vi "Dashboard Main.vi"() -> ()   [LabVIEW 2013]
uses:
  frc 2014 Vision Prototype/TargetType.ctl
  <vilib>/event_ctls.llb/eventvkey.ctl
  <vilib>/Analysis/baseanly.llb/Mean (DBL).vi
  <vilib>/Rock Robotics/WPI/Dashboard/WPI_DashboardLogging Global.vi
  <vilib>/Utility/config.llb/Write Key (String).vi
  <vilib>/Utility/config.llb/Write Key (I32).vi
  <vilib>/Utility/config.llb/NI_LVConfig.lvlib
  <vilib>/Analysis/NI_AALBase.lvlib
panel:
  out "Camera IP":string="10.15.72.11"
  out "Raw Distance":dbl[](array[numeric]) format="%#.4g"
  out "Error":bool
  out "Mask":T1(plugin-control)
  out "Target Info":T3(array[cluster])
  in  "Camera Type":enum16{"206", "1011", "1013"}(ring)=enum."1011"
  in  "Std Devs":cluster{"Hue":dbl, "Sat":dbl, "Val":dbl}={"Hue"=4.0, "Sat"=6.0, "Val"=4.0}
  out "x":dbl
  in  "Vision_Control":u8(slide) scale=0.0..2.0
  in  "Camera Settings":T4={"Frame Rate"=30, "Compression"=30, "Size"=1} {"Frame Rate" scale=1.0..30.0; "Size" items=["640x480", "320x240", "160x120"]}
  out "Image Message":string="Timeout in Camera Communications"
  in  "Rec Mode":enum32{"Stop", "Record", "Playback"}(radio)
  in  "Dashboard Tab":T5(tab)
  out "MotorSliders R":cluster{"MotorSlide1":dbl, "MotorSlide2":dbl} {"MotorSlide2" scale=-1.0..1.0 scale format="%#_2e"; "MotorSlide1" scale=-1.0..1.0 scale format="%#_2e"}
  out "MotorChart R":cluster{"Numeric":dbl, "Numeric":dbl}(graph)
  out "MotorSliders L":T6 {"MotorSlide4 2" scale=0.0..14.0 scale format="%#_2e"; "MotorSlide2" scale=-1.0..1.0 scale format="%#_2e"; "MotorSlide1" scale=-1.0..1.0 scale format="%#_2e"}
  out "MotorChart L":T7(graph)
  out "JS1 Z":dbl(slide) scale=-1.0..1.0 scale format="%#_2e"
  out "Joystick 1":cluster{"X":dbl, "Y":dbl}[](graph)
  out "JS Buttons 1":T8
  out "JS2 Z":dbl(slide) scale=-1.0..1.0 scale format="%#_2e"
  out "Joystick 2":cluster{"X":dbl, "Y":dbl}[](graph)
  out "JS Buttons 2":T8
  out "Mode":T9(ring)=enum."Auto Disabled"
  in  "DB Camera Config":bool
  out "fps":dbl format="%#.1g"
  out "Mbps":dbl format="%#.1g"
  out "Mbps 2":bool
  out "LED 1":bool
  out "Compressor_Running":bool
  out "Shooter_State":string
  out "Hot_Target_Angle":dbl(knob) scale=-90.0..90.0
  out "Target_Left_Hot":bool
  out "units 2":string="feet"
  out "vision_target_distance":dbl(slide) caption="sonar_distance" scale=0.0..25.0 scale format="%#.3g"
  out "units":string="inches"
  out "sonar_ball_distance":dbl(slide) caption="sonar_distance" scale=0.0..120.0 scale format="%#.3g"
  out "robot_heading":dbl(knob) scale=0.0..360.0
  out "Target_Right_Hot":bool
  in  "Dist_Fifo":i32=5
  in  "Color Components":T10={"Hue"={100.0, 190.0}, "Sat"={121.42857142857142, 255.0}, "Val"={188.2142857142857, 255.0}} {"Val" scale=0.0..255.0; "Sat" scale=0.0..255.0; "Hue" scale=0.0..255.0 scale format="%#_3g"}
  in  "Area Size Limit %":dbl=0.06 format="%#_13g"
  in  "Score Cutoff":dbl(slide)=54.248366013071895 scale=0.0..100.0
  in  "Fudge Factor":dbl=-1.0
  in  "Scale Factor Adustment":dbl
  out "Median \nDistance":dbl
  out "Final Target Dist From Center":dbl
  out "Final Target\nDistance":dbl
  in  "Test Slider":dbl(slide) scale=0.0..100.0 scale format="%#_3g"
  in  "On/Off":bool caption="Solenoid"
  in  "Test Name":u16(ring) items=["Select the test to run...", "Example Test", "-------------------------------", "List of tests is built in robot code.", "Replace with your own automated tests."]
  in  "Test Tree":string(tree)
  in  "Motor":cluster{"Value":dbl, "Enable":bool} {"Value" scale=-1.0..1.0 scale format="%#_3g"}
  out "Progress":T11 {"Test Progress" scale=0.0..100.0}
  in  "Rev/Fwd":cluster{"Forward":bool, "Reverse":bool}
  in  "Test Ring":u16(ring) items=["Auto", "Fixed indoor", "Fixed outdoor 1", "Fixed outdoor 2", "Fixed fluorescent 1", "Fixed fluorescent 2", "Hold current"]
  in  "Listbox":i32(listbox)
  out "Tree":string(tree)
  out "Camera Image":T1(plugin-control)
  # "Left"
  # "Front"
  # "Right"
  # "Battery"
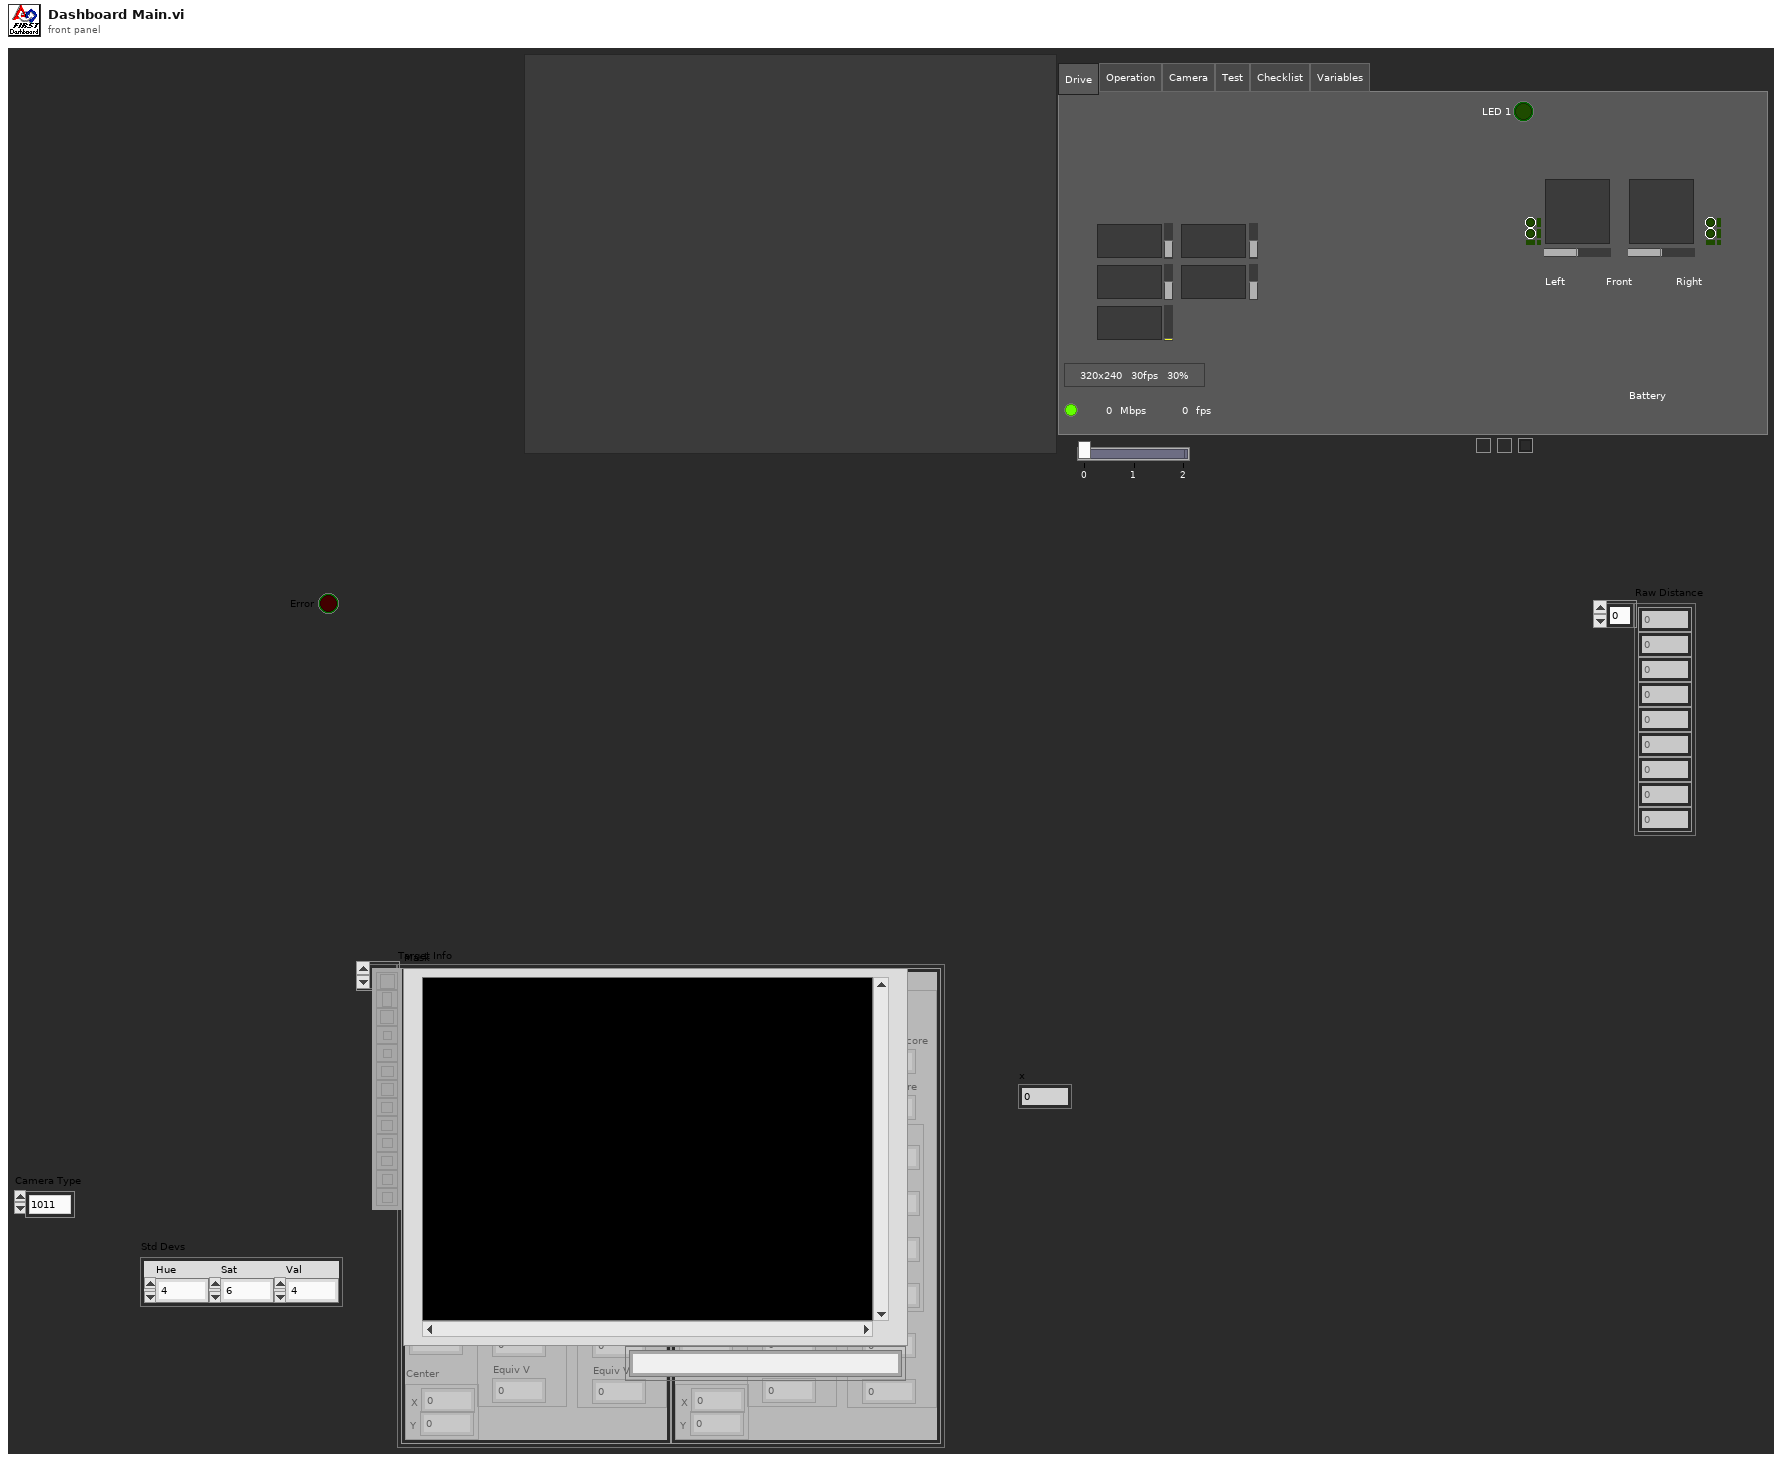
[diagram p1: front panel]
types:
  T1 = typedef "IMAQ Image.ctl" = refnum<image>
  T2 = typedef "TargetType.ctl" = enum16{"Not Hot", "Hot"}
  T3 = cluster{"Scores":cluster{"Total":dbl, "Left":dbl, "Right":dbl, "Ratio":dbl, "Vertical":dbl, "index":i32, "State":T2}, "Verticals":cluster{"Horizontal?":bool, "Aspect Score":dbl, "Rect Score":dbl, cluster{"Left":dbl, "Top":dbl, "Right":dbl, "Bottom":dbl}, "Equiv H":dbl, "Equiv V":dbl}, "Horizontals":cluster{"Horizontal?":bool, "Aspect Score":dbl, "Rect Score":dbl, cluster{"Left":dbl, "Top":dbl, "Right":dbl, "Bottom":dbl}, "Equiv H":dbl, "Equiv V":dbl}, "Distance ft":dbl, "Center":cluster{"X":dbl, "Y":dbl}}[]
  T4 = cluster{"Frame Rate":i32, "Compression":i32, "Size":u16}
  T5 = enum32{"Drive", "Operation", "Camera", "Test", "Checklist", "Variables"}
  T6 = cluster{"MotorSlide1":dbl, "MotorSlide2":dbl, "MotorSlide4 2":dbl}
  T7 = cluster{"Numeric":dbl, "Numeric":dbl, "Battery":sgl}
  T8 = cluster{bool, bool, bool, bool, bool, bool, bool, bool, bool, bool, bool, bool}
  T9 = enum8{"Tele-Op Disabled", "Tele-Op Enabled", "Auto Disabled", "Auto Enabled", "Test Disabled", "Test Enabled", ""}
  T10 = cluster{"Hue":cluster{dbl, dbl}, "Sat":cluster{dbl, dbl}, "Val":cluster{dbl, dbl}}
  T11 = cluster{"Test Progress":u8, "Test Progress Text":string}
  T12 = enum32{"Drive", "Operation", "Auto", "Test", "Checklist", "Variables"}
  T13 = typedef "Image Type" = u32
  T14 = cluster{"Horizontal":bool, "Aspect Score":dbl, "Rect Score":dbl, cluster{"Left":dbl, "Top":dbl, "Right":dbl, "Bottom":dbl}, "Equiv H":dbl, "Equiv V":dbl}[]
  T15 = cluster{cluster{dbl, dbl}, cluster{dbl, dbl}, cluster{dbl, dbl}}
  T16 = cluster{"Scores":cluster{"Total":dbl, "Left":dbl, "Right":dbl, "Ratio":dbl, "Vertical":dbl, "index":i32, "State":T2}, "Verticals":cluster{"Horizontal?":bool, "Aspect Score":dbl, "Rect Score":dbl, cluster{"Left":dbl, "Top":dbl, "Right":dbl, "Bottom":dbl}, "Equiv H":dbl, "Equiv V":dbl}, "Horizontals":cluster{"Horizontal?":bool, "Aspect Score":dbl, "Rect Score":dbl, cluster{"Left":dbl, "Top":dbl, "Right":dbl, "Bottom":dbl}, "Equiv H":dbl, "Equiv V":dbl}, "Validated":bool}[]
  T17 = cluster{"Distance (ft)":dbl, "Target Center (-1 to 1)":cluster{"X":dbl, "Y":dbl}, "Left":bool, "State":T2}[]
  T18 = cluster{"Scores":cluster{"Total":dbl, "Left":dbl, "Right":dbl, "Ratio":dbl, "Vertical":dbl, "index":i32, "State":T2}, "Verticals":cluster{"Horizontal?":bool, "Aspect Score":dbl, "Rect Score":dbl, cluster{"Left":dbl, "Top":dbl, "Right":dbl, "Bottom":dbl}, "Equiv H":dbl, "Equiv V":dbl}, "Horizontals":cluster{"Horizontal?":bool, "Aspect Score":dbl, "Rect Score":dbl, cluster{"Left":dbl, "Top":dbl, "Right":dbl, "Bottom":dbl}, "Equiv H":dbl, "Equiv V":dbl}, "Distance (ft)":dbl, "Target Center (-1 to 1)":cluster{"X":dbl, "Y":dbl}}[]
  T19 = cluster{"Distances[0]":cluster{"Distance (ft)":dbl, "Target Center (-1 to 1)":cluster{"X":dbl, "Y":dbl}, "Left":bool, "State":T2}, "Distances[1]":cluster{"Distance (ft)":dbl, "Target Center (-1 to 1)":cluster{"X":dbl, "Y":dbl}, "Left":bool, "State":T2}, "Distances[2]":cluster{"Distance (ft)":dbl, "Target Center (-1 to 1)":cluster{"X":dbl, "Y":dbl}, "Left":bool, "State":T2}, "Distances[3]":cluster{"Distance (ft)":dbl, "Target Center (-1 to 1)":cluster{"X":dbl, "Y":dbl}, "Left":bool, "State":T2}, "Distances[4]":cluster{"Distance (ft)":dbl, "Target Center (-1 to 1)":cluster{"X":dbl, "Y":dbl}, "Left":bool, "State":T2}, "Distances[5]":cluster{"Distance (ft)":dbl, "Target Center (-1 to 1)":cluster{"X":dbl, "Y":dbl}, "Left":bool, "State":T2}, "Distances[6]":cluster{"Distance (ft)":dbl, "Target Center (-1 to 1)":cluster{"X":dbl, "Y":dbl}, "Left":bool, "State":T2}, "Distances[7]":cluster{"Distance (ft)":dbl, "Target Center (-1 to 1)":cluster{"X":dbl, "Y":dbl}, "Left":bool, "State":T2}, "Distances[8]":cluster{"Distance (ft)":dbl, "Target Center (-1 to 1)":cluster{"X":dbl, "Y":dbl}, "Left":bool, "State":T2}}
  T20 = cluster{"Target Info[0]":cluster{"Scores":cluster{"Total":dbl, "Left":dbl, "Right":dbl, "Ratio":dbl, "Vertical":dbl, "index":i32, "State":T2}, "Verticals":cluster{"Horizontal?":bool, "Aspect Score":dbl, "Rect Score":dbl, cluster{"Left":dbl, "Top":dbl, "Right":dbl, "Bottom":dbl}, "Equiv H":dbl, "Equiv V":dbl}, "Horizontals":cluster{"Horizontal?":bool, "Aspect Score":dbl, "Rect Score":dbl, cluster{"Left":dbl, "Top":dbl, "Right":dbl, "Bottom":dbl}, "Equiv H":dbl, "Equiv V":dbl}, "Distance (ft)":dbl, "Target Center (-1 to 1)":cluster{"X":dbl, "Y":dbl}}, "Target Info[1]":cluster{"Scores":cluster{"Total":dbl, "Left":dbl, "Right":dbl, "Ratio":dbl, "Vertical":dbl, "index":i32, "State":T2}, "Verticals":cluster{"Horizontal?":bool, "Aspect Score":dbl, "Rect Score":dbl, cluster{"Left":dbl, "Top":dbl, "Right":dbl, "Bottom":dbl}, "Equiv H":dbl, "Equiv V":dbl}, "Horizontals":cluster{"Horizontal?":bool, "Aspect Score":dbl, "Rect Score":dbl, cluster{"Left":dbl, "Top":dbl, "Right":dbl, "Bottom":dbl}, "Equiv H":dbl, "Equiv V":dbl}, "Distance (ft)":dbl, "Target Center (-1 to 1)":cluster{"X":dbl, "Y":dbl}}, "Target Info[2]":cluster{"Scores":cluster{"Total":dbl, "Left":dbl, "Right":dbl, "Ratio":dbl, "Vertical":dbl, "index":i32, "State":T2}, "Verticals":cluster{"Horizontal?":bool, "Aspect Score":dbl, "Rect Score":dbl, cluster{"Left":dbl, "Top":dbl, "Right":dbl, "Bottom":dbl}, "Equiv H":dbl, "Equiv V":dbl}, "Horizontals":cluster{"Horizontal?":bool, "Aspect Score":dbl, "Rect Score":dbl, cluster{"Left":dbl, "Top":dbl, "Right":dbl, "Bottom":dbl}, "Equiv H":dbl, "Equiv V":dbl}, "Distance (ft)":dbl, "Target Center (-1 to 1)":cluster{"X":dbl, "Y":dbl}}, "Target Info[3]":cluster{"Scores":cluster{"Total":dbl, "Left":dbl, "Right":dbl, "Ratio":dbl, "Vertical":dbl, "index":i32, "State":T2}, "Verticals":cluster{"Horizontal?":bool, "Aspect Score":dbl, "Rect Score":dbl, cluster{"Left":dbl, "Top":dbl, "Right":dbl, "Bottom":dbl}, "Equiv H":dbl, "Equiv V":dbl}, "Horizontals":cluster{"Horizontal?":bool, "Aspect Score":dbl, "Rect Score":dbl, cluster{"Left":dbl, "Top":dbl, "Right":dbl, "Bottom":dbl}, "Equiv H":dbl, "Equiv V":dbl}, "Distance (ft)":dbl, "Target Center (-1 to 1)":cluster{"X":dbl, "Y":dbl}}, "Target Info[4]":cluster{"Scores":cluster{"Total":dbl, "Left":dbl, "Right":dbl, "Ratio":dbl, "Vertical":dbl, "index":i32, "State":T2}, "Verticals":cluster{"Horizontal?":bool, "Aspect Score":dbl, "Rect Score":dbl, cluster{"Left":dbl, "Top":dbl, "Right":dbl, "Bottom":dbl}, "Equiv H":dbl, "Equiv V":dbl}, "Horizontals":cluster{"Horizontal?":bool, "Aspect Score":dbl, "Rect Score":dbl, cluster{"Left":dbl, "Top":dbl, "Right":dbl, "Bottom":dbl}, "Equiv H":dbl, "Equiv V":dbl}, "Distance (ft)":dbl, "Target Center (-1 to 1)":cluster{"X":dbl, "Y":dbl}}, "Target Info[5]":cluster{"Scores":cluster{"Total":dbl, "Left":dbl, "Right":dbl, "Ratio":dbl, "Vertical":dbl, "index":i32, "State":T2}, "Verticals":cluster{"Horizontal?":bool, "Aspect Score":dbl, "Rect Score":dbl, cluster{"Left":dbl, "Top":dbl, "Right":dbl, "Bottom":dbl}, "Equiv H":dbl, "Equiv V":dbl}, "Horizontals":cluster{"Horizontal?":bool, "Aspect Score":dbl, "Rect Score":dbl, cluster{"Left":dbl, "Top":dbl, "Right":dbl, "Bottom":dbl}, "Equiv H":dbl, "Equiv V":dbl}, "Distance (ft)":dbl, "Target Center (-1 to 1)":cluster{"X":dbl, "Y":dbl}}, "Target Info[6]":cluster{"Scores":cluster{"Total":dbl, "Left":dbl, "Right":dbl, "Ratio":dbl, "Vertical":dbl, "index":i32, "State":T2}, "Verticals":cluster{"Horizontal?":bool, "Aspect Score":dbl, "Rect Score":dbl, cluster{"Left":dbl, "Top":dbl, "Right":dbl, "Bottom":dbl}, "Equiv H":dbl, "Equiv V":dbl}, "Horizontals":cluster{"Horizontal?":bool, "Aspect Score":dbl, "Rect Score":dbl, cluster{"Left":dbl, "Top":dbl, "Right":dbl, "Bottom":dbl}, "Equiv H":dbl, "Equiv V":dbl}, "Distance (ft)":dbl, "Target Center (-1 to 1)":cluster{"X":dbl, "Y":dbl}}, "Target Info[7]":cluster{"Scores":cluster{"Total":dbl, "Left":dbl, "Right":dbl, "Ratio":dbl, "Vertical":dbl, "index":i32, "State":T2}, "Verticals":cluster{"Horizontal?":bool, "Aspect Score":dbl, "Rect Score":dbl, cluster{"Left":dbl, "Top":dbl, "Right":dbl, "Bottom":dbl}, "Equiv H":dbl, "Equiv V":dbl}, "Horizontals":cluster{"Horizontal?":bool, "Aspect Score":dbl, "Rect Score":dbl, cluster{"Left":dbl, "Top":dbl, "Right":dbl, "Bottom":dbl}, "Equiv H":dbl, "Equiv V":dbl}, "Distance (ft)":dbl, "Target Center (-1 to 1)":cluster{"X":dbl, "Y":dbl}}, "Target Info[8]":cluster{"Scores":cluster{"Total":dbl, "Left":dbl, "Right":dbl, "Ratio":dbl, "Vertical":dbl, "index":i32, "State":T2}, "Verticals":cluster{"Horizontal?":bool, "Aspect Score":dbl, "Rect Score":dbl, cluster{"Left":dbl, "Top":dbl, "Right":dbl, "Bottom":dbl}, "Equiv H":dbl, "Equiv V":dbl}, "Horizontals":cluster{"Horizontal?":bool, "Aspect Score":dbl, "Rect Score":dbl, cluster{"Left":dbl, "Top":dbl, "Right":dbl, "Bottom":dbl}, "Equiv H":dbl, "Equiv V":dbl}, "Distance (ft)":dbl, "Target Center (-1 to 1)":cluster{"X":dbl, "Y":dbl}}}
  T21 = cluster{"Horizontal?":bool, "Aspect Score":dbl, "Rect Score":dbl, cluster{"Left":dbl, "Top":dbl, "Right":dbl, "Bottom":dbl}, "Equiv H":dbl, "Equiv V":dbl}
  T22 = cluster{"Left":dbl, "Top":dbl, "Right":dbl, "Bottom":dbl}
  T23 = cluster{"Distance (ft)":dbl, "Left":dbl, "Right":dbl}
  T24 = cluster{"Digital Inputs":bool[], "Digital Outputs":bool[]}
  T25 = cluster{"Competition mode":bool, "Robot Link":bool, "Autonomous":bool, "Enabled":bool, "E-Stop":bool, "Simulated":bool, "TestMode":bool, "Docked Window":bool}
  T26 = cluster{"Boolean Array[0]":bool, "Boolean Array[1]":bool, "Boolean Array[2]":bool, "Boolean Array[3]":bool, "Boolean Array[4]":bool, "Boolean Array[5]":bool, "Boolean Array[6]":bool, "Boolean Array[7]":bool, "Boolean Array[8]":bool, "Boolean Array[9]":bool, "Boolean Array[10]":bool, "Boolean Array[11]":bool}
  T27 = typedef "NI_LVConfig.lvlib/Config Data RefNum.ctl" = refnum<k1>
  T28 = typedef "eventvkey.ctl" = enum16{"ASCII", "Enter", "Return", "Shift", "Ctrl", "Alt", "Cmd", "Opt", "Caps", "NumLock", "Clear", "Break", "Up", "Down", "Left", "Right", "Insert", "Delete", "Home", "End", "PageUp", "PageDown", "Escape", "Help", "Pause", "ScrollLock", "F1", "F2", "F3", "F4", "F5", "F6", "F7", "F8", "F9", "F10", "F11", "F12", "F13", "F14", "F15", "F16", "F17", "F18", "F19", "F20", "F21", "F22", "F23", "F24", "Play", "VolumeUp", "VolumeDown", "Mute", "Two Byte Char"}
  T29 = cluster{"Image Size":bool, "Image Type":bool, "Pixel Value":bool, "ROI Information":bool, "Zoom Factor":bool}
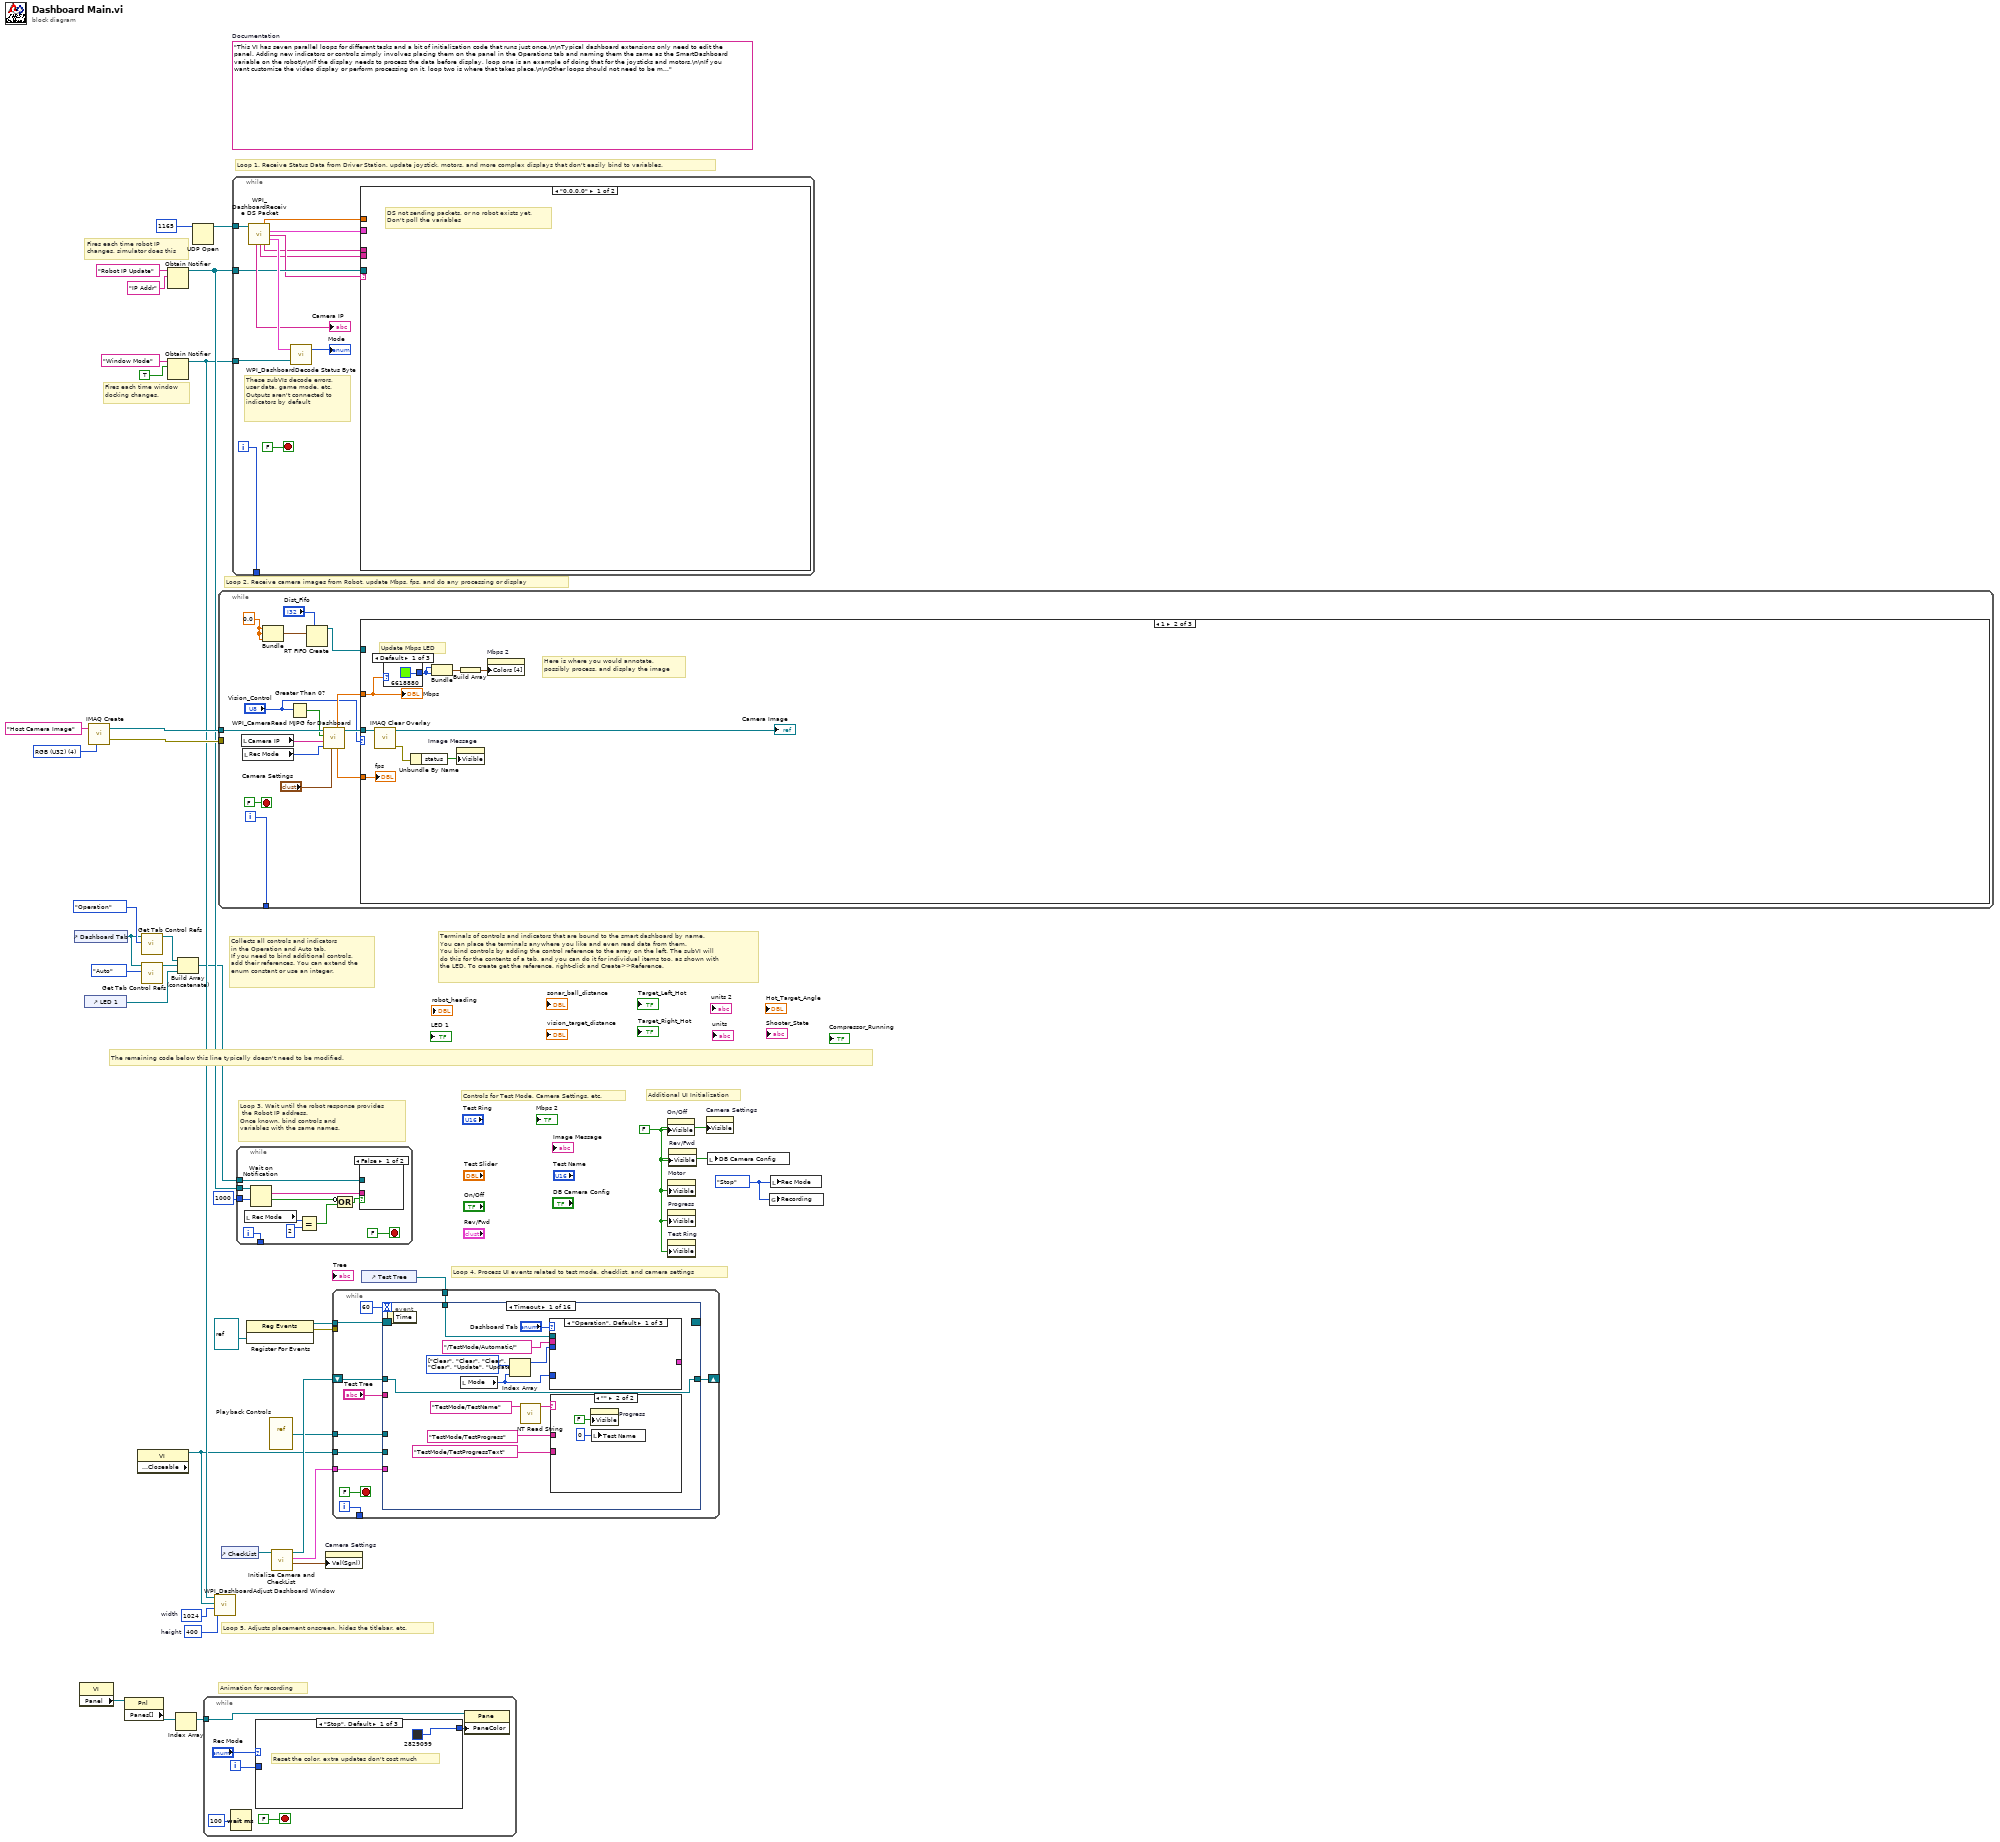
[diagram p0: block diagram]
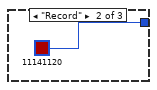
[diagram p2: hidden frame]
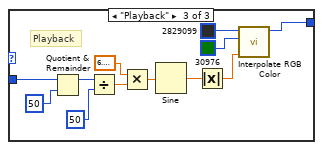
[diagram p3: hidden frame]
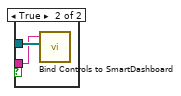
[diagram p4: hidden frame]
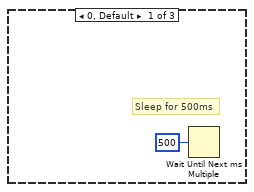
[diagram p5: hidden frame]
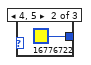
[diagram p6: hidden frame]
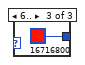
[diagram p7: hidden frame]
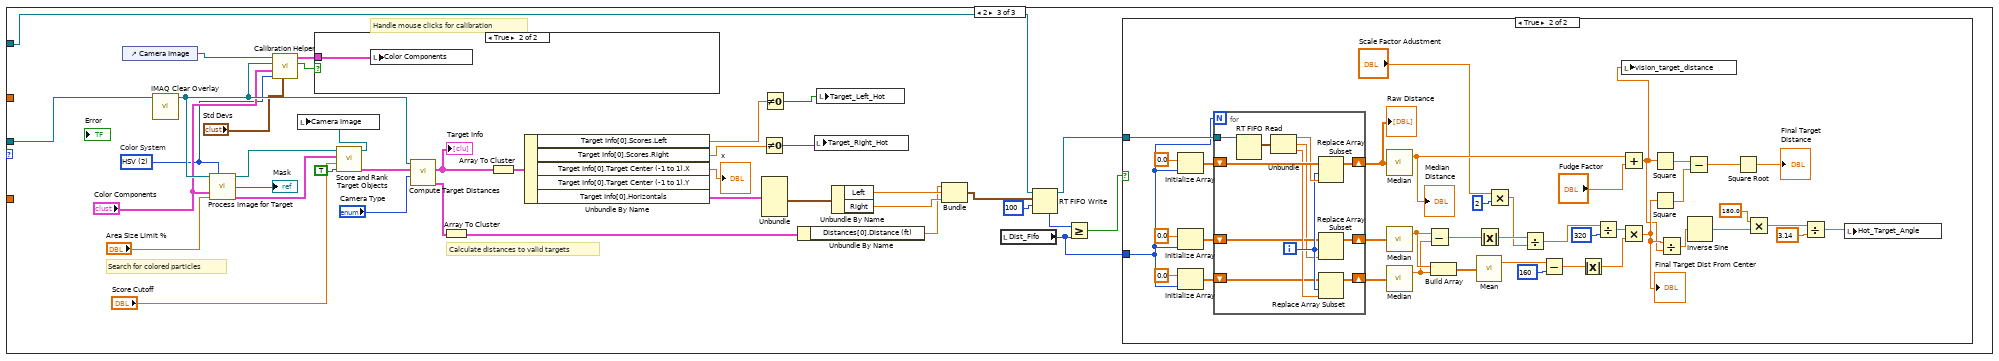
[diagram p8: hidden frame]
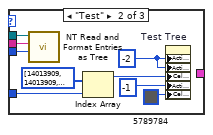
[diagram p11: hidden frame]
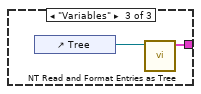
[diagram p12: hidden frame]
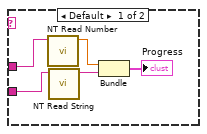
[diagram p13: hidden frame]
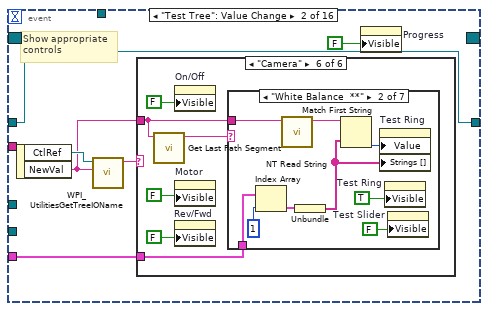
[diagram p14: hidden frame]
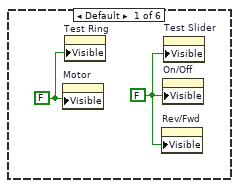
[diagram p15: hidden frame]
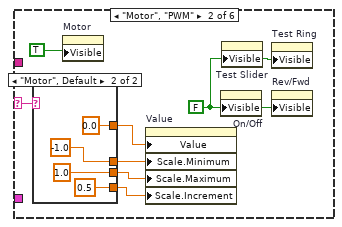
[diagram p16: hidden frame]
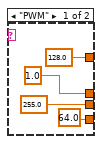
[diagram p17: hidden frame]
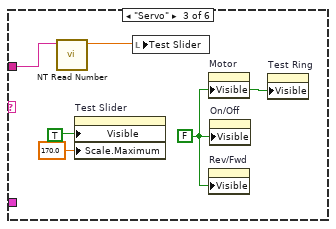
[diagram p18: hidden frame]
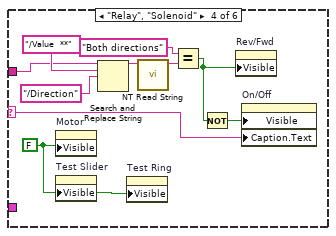
[diagram p19: hidden frame]
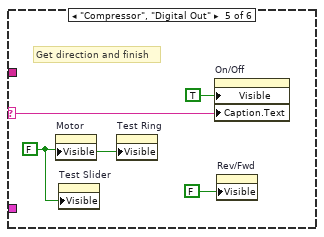
[diagram p20: hidden frame]
diagram:
  w8 = enum32{"Stop", "Record", "Playback"}."Stop" ("Rec Mode")
  w11 = 400  # height
  w12 = 1024  # width
  w25 = FALSE ("Visible")
  (unwired) "This VI has seven parallel loops for different tasks and a bit of initialization code that runs just once.\n\nTypical dashboard extensions only need to edit the panel. Adding new indicators or controls simply involves placing them on the panel in the Operations tab and naming them the same as the SmartDashboard variable on the robot\n\nIf the display needs to process the data before display, loop one is an example of doing that for the joysticks and motors.\n\nIf you want customize the video display or perform processing on it, loop two is where that takes place.\n\nOther loops should not need to be modified. They are pretty standard, and document the task they perform."  # Documentation
  w35 = T13 4 items=["Grayscale (U8)", "Grayscale (I16)", "Grayscale (SGL)", "Complex (CSG)", "RGB (U32)", "HSL (U32)", "RGB (U64)"] ("Image Type")
  # "Controls for Test Mode, Camera Settings, etc."
  # "Additional UI Initialization"
  # "Animation for recording"
  # "Fires each time robot IP\nchanges, simulator does this"
  # "Fires each time window\ndocking changes."
  # "Collects all controls and indicators\nin the Operation and Auto tab.\nIf you need to bind additional controls,\nadd their references. You can extend the\nenum constant or use an integer."
  # "The remaining code below this line typically doesn't need to be modified."
  # "Loop 4. Process UI events related to test mode, checklist, and camera settings"
  # "Terminals of controls and indicators that are bound to the smart dashboard by name.\nYou can place the terminals anywhere you like and even read data from them.\nYou bind controls by adding the control reference to the array on the left. The subVI will\ndo this for the contents of a tab, and you can do it for individual items too, as shown with\nthe LED. To create get the reference, right-click and Create>>Reference."
  # "Loop 3. Wait until the robot response provides\n the Robot IP address.\nOnce known, bind controls and\nvariables with the same names."
  # "Loop 5. Adjusts placement onscreen, hides the titlebar, etc."
  # "Loop 1. Receive Status Data from Driver Station, update joystick, motors, and more complex displays that don't easily bind to variables."
  # "Loop 2. Receive camera images from Robot, update Mbps, fps, and do any processing or display"
  n1 = control-ref of="Dashboard Tab"() -> (w6:refnum<vi>)
  n2 = property class="VI"() -> ("Panel"=w19:refnum<vi>)  [unwired: 2 in, 2 out]
  n3 = control-ref of="LED 1"() -> (w1:refnum<vi>)
  n4 = call "IMAQ Create"("Image Name"="Host Camera Image", "Image Type"=w35) -> ("New Image"=w33:T1, "error out"=w32:errorcluster)  [unwired: 2 in, 1 out]
  n5 = property class="Pnl"(reference=w19) -> ("Panes[]"=w20:refnum<vi>[])  [unwired: 1 in, 2 out]
  n6 = property class="VI" props=["Front Panel.Closeable"]() -> (reference out=w7:refnum<vi>)  [unwired: 2 in, 2 out]
  n7 = call <vilib>:"Get Tab Control Refs.vi"("Page Index"=T12."Operation" ("Dashboard Tab"), "TabControl in"=w6) -> ("ControlsOnPage"=w4:refnum<vi>[])  [unwired: 9 in]
  n8 = call <vilib>:"Get Tab Control Refs.vi"("Page Index"=T12."Auto" ("Dashboard Tab"), "TabControl in"=w6) -> ("ControlsOnPage"=w5:refnum<vi>[])  [unwired: 9 in]
  n9 = Obtain Notifier(name (unnamed)="Robot IP Update", notification data type="IP Addr" ("name (unnamed)")) -> (notifier out=w29:refnum<notifier>)  [unwired: 2 in, 2 out]
  n10 = Obtain Notifier(name (unnamed)="Window Mode", notification data type=TRUE) -> (notifier out=w10:refnum<notifier>)  [unwired: 2 in, 2 out]
  n11 = Index Array(array=w20) -> (element=w18:refnum<vi>)  [unwired: 1 in]
  n12 = Build Array (concatenate)(w4, w5, w1) -> (w3:refnum<vi>[])
  n13 = UDP Open(11:u16 1165 ("port")) -> (port=w36:refnum<k16>)  [unwired: 2 in, 4 out]
  n14 = while {
    tunnel: w18 -> [w39]
    i -> [w42]
    stop <- FALSE stop-if-true
    n15 = Wait (ms)(milliseconds to wait=u32 100) -> ()  [unwired: 1 out]
    n16 = case shown="\"Stop\", Default" "Rec Mode" {
      tunnel: w42 -> [_ _ w57]
      tunnel: [u32 2829099 ("Base Color") u32 11141120 ("Target Color") w46] -> w38
      frame "Stop", Default {
        # "Reset the color, extra updates don't cost much"
      }
      frame "Record" {
      }
      frame "Playback" {
        # "Playback"
        n17 = Quotient & Remainder(x=w57, y=u32 50 ("milliseconds to wait")) -> (x-y*floor(x/y)=w53:u32)  [unwired: 1 out]
        n18 = Divide(x=w53, y=u32 50 ("milliseconds to wait")) -> (x/y=w50:dbl)
        n19 = Multiply(x=6.283185307179586, y=w50) -> (x*y=w55:dbl)
        n20 = Sine(x=w55) -> (sin(x)=w54:dbl)
        n21 = Absolute Value(x=w54) -> (abs(x)=w47:dbl)
        n22 = call "Interpolate RGB Color.vi"("Proportion"=w47, "Target Color"=u32 30976, "Base Color"=u32 2829099) -> ("Result Color"=w46:u32)  [unwired: 8 in]
      }
    }
    n23 = property class="Pane"(reference=w39, "PaneColor"=w38) -> ()  [unwired: 1 in, 2 out]
  }
  n24 = call <vilib>:"WPI_DashboardAdjust Dashboard Window.vi"("height"=w11, "width"=w12, "reference in"=w7, "Notifier in"=w10) -> ()  [unwired: 8 in]
  n25 = while {
    tunnel: w33 -> [w70]
    tunnel: w32 -> [_]
    tunnel: [w71] -> _
    i -> [w71]
    stop <- FALSE stop-if-true
    w61 = 0.0
    n26 = local read "Camera IP"() -> (w65:string)
    n27 = local read "Rec Mode"() -> (w64:enum32{"Stop", "Record", "Playback"})
    n28 = Bundle(w61, w61, w61) -> (w60:cluster{dbl, dbl, dbl})  [unwired: 1 in]
    n29 = Greater Than 0?(x="Vision_Control") -> (x > 0?=w63:bool)
    n30 = RT FIFO Create(1:w60, 4:"Dist_Fifo") -> (8:w58:refnum<k33>)  [unwired: 6 in, 2 out]
    n31 = call <vilib>:"WPI_CameraRead MJPG for Dashboard.vi"("Camera Settings"="Camera Settings", "Rec Mode"=w64, "Camera IP"=w65, "Enable"=w63, "Refnum in"=w70) -> ("Refnum out"=w69:T1, "FPS"=w68:dbl, "Bandwidth (Mbps)"=w67:dbl)  [unwired: 3 in, 1 out]
    n32 = case shown="1" "Vision_Control" {
      tunnel: w69 -> [_ w77 w97]
      tunnel: w67 -> [_ w76 _]
      tunnel: w68 -> [_ w74 _]
      tunnel: w58 -> [_ _ w92]
      frame 0, Default {
        # "Sleep for 500ms"
        n33 = Wait Until Next ms Multiple(millisecond multiple=u32 500) -> ()  [unwired: 1 out]
      }
      frame 1 {
        # "Here is where you would annotate,\npossibly process, and display the image"
        # "Update Mbps LED"
        n34 = call "IMAQ Clear Overlay"("Image"=w77) -> ("error out"=w81:errorcluster, "Image Out"=→"Camera Image":T1)  [unwired: 2 in, 7 out]
        n35 = case shown="Default" w76 {
          tunnel: [u32 6618880 ("Color Box") u32 16776722 ("Color Box") u32 16716800 ("Color Box")] -> w78
          frame Default {
          }
          frame 4, 5 {
          }
          frame 6.. {
          }
        }
        n36 = Unbundle By Name(w81) -> ("status"=w82:bool)
        n37 = Bundle("Color Box"=w78, "Color Box"=w78) -> (w80:cluster{"Color Box":u32, "Color Box":u32})  [unwired: 1 out]
        n38 = property on="Image Message" class="Str"("Visible"=w82) -> ()  [unwired: 2 in, 2 out]
        n39 = Build Array(w80) -> (w79:cluster{"Color Box":u32, "Color Box":u32}[])
        n40 = property on="Mbps 2" class="Bool (strict)"("Colors [4]"=w79) -> ()  [unwired: 2 in, 2 out]
        "Mbps" <- w76
        "fps" <- w74
      }
      frame 2 {
        w105 = u16 2 items=["RGB", "HSL", "HSV", "HSI"]  # Color System
        # "Calculate distances to valid targets"
        # "Search for colored particles"
        # "Handle mouse clicks for calibration"
        n41 = control-ref of="Camera Image"() -> (w96:refnum<vi>)
        n42 = call "IMAQ Clear Overlay"("Image"=w97) -> ("Image Out"=w110:T1)  [unwired: 9 in, 1 out]
        n43 = call "Process Image for Target.vi"("Src Image"=w110, "Color Mode"=w105, "Color Components"="Color Components", "Area Cutoff %"="Area Size Limit %") -> ("Src Image Out"=w101:T1, "Threshold"=→"Mask":T1, "Particles"=w102:T14)  [unwired: 9 in]
        n44 = call "Calibration Helper.vi"("Std Devs"="Std Devs", "Color Mode"=w105, "Color Components"="Color Components", "Image"=w110, "Image Ctl Refnum"=w96) -> ("Changed"=w109:bool, "output color"=w107:T15)  [unwired: 5 in]
        n45 = case shown="True" w109 {
          tunnel: w107 -> [_ w176]
          frame False {
          }
          frame True {
            n46 = local write "Color Components"(w176) -> ()
          }
        }
        n47 = call "Score and Rank Target Objects.vi"("Annotate"=TRUE, "Score Limit"="Score Cutoff", "Particles"=w102, "Image in"=w101) -> ("Target Info"=w103:T16, "Annotated Image"=w86:T1)  [unwired: 6 in]
        n48 = local write "Camera Image"(w86) -> ()
        n49 = call "Compute Target Distances.vi"("Camera Type"="Camera Type", "Target Info"=w103, "Image in"=w110) -> ("Distances"=w112:T17, "Target Info"=w117:T18)  [unwired: 6 in, 1 out]
        "Target Info" <- w117
        n50 = Array To Cluster(array=w112) -> (cluster=w113:T19)
        n51 = Array To Cluster(array=w117) -> (cluster=w116:T20)
        n52 = Unbundle By Name(w116) -> ("Target Info[0].Scores.Left"=w115:dbl, "Target Info[0].Scores.Right"=w114:dbl, "Target Info[0].Target Center (-1 to 1).X"=→"x":dbl, "Target Info[0].Horizontals"=w119:T21)  [unwired: 1 out]
        n53 = Not Equal To 0?(x=w114) -> (x != 0?=w87:bool)
        n54 = Unbundle(w119) -> (w120:T22)  [unwired: 5 out]
        n55 = Not Equal To 0?(x=w115) -> (x != 0?=w88:bool)
        n56 = Unbundle By Name(w113) -> ("Distances[0].Distance (ft)"=w121:dbl)
        n57 = local write "Target_Right_Hot"(w87) -> ()
        n58 = local write "Target_Left_Hot"(w88) -> ()
        n59 = Unbundle By Name(w120) -> ("Left"=w123:dbl, "Right"=w122:dbl)
        n60 = Bundle("Distance (ft)"=w121, "Left"=w123, "Right"=w122) -> (w93:T23)  [unwired: 1 in]
        n61 = local read "Dist_Fifo"() -> (w89:i32)
        n62 = RT FIFO Write(0:w92, 1:w93, 2:100) -> (7:w94:u32, 8:w91:refnum<k33>)  [unwired: 2 in, 2 out]
        n63 = Greater Or Equal?(x=w94, y=w89) -> (x >= y?=w90:bool)
        n64 = case shown="True" w90 {
          tunnel: w91 -> [_ w163]
          tunnel: w89 -> [_ w127]
          frame False {
          }
          frame True {
            n65 = Initialize Array(0.0, w127) -> (w161:dbl[])
            n66 = Initialize Array(0.0, w127) -> (w146:dbl[])
            n67 = Initialize Array(0.0, w127) -> (w145:dbl[])
            n68 = for {
              N: w127 -> [_]
              shift-right: [w173] -> w160
              shift-left: w161 -> [w174]
              tunnel: w163 -> [w175]
              shift-right: [w167] -> w144
              shift-left: w146 -> [w168]
              shift-right: [w165] -> w143
              shift-left: w145 -> [w166]
              i -> [w170]
              n69 = RT FIFO Read(0:w175) -> (9:w172:cluster{dbl, dbl, dbl})  [unwired: 3 in, 4 out]
              n70 = Unbundle(w172) -> (w171:dbl, w164:dbl, w169:dbl)
              n71 = Replace Array Subset(array=w174, new element=w171, index=w170) -> (w173:dbl[])
              n72 = Replace Array Subset(array=w168, new element=w164, index=w170) -> (w167:dbl[])
              n73 = Replace Array Subset(array=w166, new element=w169, index=w170) -> (w165:dbl[])
            }
            "Raw Distance" <- w160
            n74 = call <vilib>:"Median.vi"("X"=w160) -> ("median"=w158:dbl)  [unwired: 1 out]
            "Median \nDistance" <- w158
            n75 = call <vilib>:"Median.vi"("X"=w144) -> ("median"=w142:dbl)  [unwired: 1 out]
            n76 = call <vilib>:"Median.vi"("X"=w143) -> ("median"=w141:dbl)  [unwired: 1 out]
            n77 = Subtract(x=w142, y=w141) -> (x-y=w157:dbl)
            n78 = Build Array(w142, w141) -> (w140:dbl[])
            n79 = call-poly <vilib>:"Mean.vi"("X"=w140) -> ("mean"=w155:dbl)  [unwired: 1 out]
            n80 = Absolute Value(x=w157) -> (abs(x)=w150:dbl)
            n81 = Multiply(x="Scale Factor Adustment", y=2) -> (x*y=w134:dbl)
            n82 = Divide(x=w150, y=w134) -> (x/y=w149:dbl)
            n83 = Subtract(x=w155, y=160) -> (x-y=w154:dbl)
            n84 = Absolute Value(x=w154) -> (abs(x)=w153:dbl)
            n85 = Divide(x=w149, y=320) -> (x/y=w151:dbl)
            n86 = Add(x=w158, y="Fudge Factor") -> (x+y=w125:dbl)
            n87 = Multiply(x=w151, y=w153) -> (x*y=w128:dbl)
            "Final Target Dist From Center" <- w128
            n88 = local write "vision_target_distance"(w125) -> ()
            n89 = Square(x=w125) -> (x^2=w137:dbl)
            n90 = Square(x=w128) -> (x^2=w138:dbl)
            n91 = Divide(x=w128, y=w125) -> (x/y=w129:dbl)
            n92 = Subtract(x=w137, y=w138) -> (x-y=w139:dbl)
            n93 = Inverse Sine(1:w129) -> (0:w130:dbl)
            n94 = Square Root(x=w139) -> (sqrt(x)=→"Final Target\nDistance":dbl)
            n95 = Multiply(x=180.0, y=w130) -> (x*y=w131:dbl)
            n96 = Divide(x=w131, y=3.14) -> (x/y=w126:dbl)
            n97 = local write "Hot_Target_Angle"(w126) -> ()
          }
        }
      }
    }
  }
  n98 = control-ref of="CheckList"() -> (w9:refnum<vi>)
  n99 = while {
    tunnel: w36 -> [w187]
    tunnel: w29 -> [w182]
    tunnel: w10 -> [w186]
    tunnel: [w183] -> _
    i -> [w183]
    stop <- FALSE stop-if-true
    # "These subVIs decode errors, user data, game mode, etc.\nOutputs aren't connected to indicators by default"
    n100 = call <vilib>:"WPI_DashboardReceive DS Packet.vi"("Recv Socket"=w187) -> ("Battery"=w177:sgl, "Driver Station"=w178:T24, "Robot IP Address"=w181:string, "Status"=w188:T25, "Camera IP Address"=→"Camera IP":string, "Low Priority User Data"=w180:string, "High Priority User Data"=w179:string)  [unwired: 1 in, 7 out]
    n101 = call <vilib>:"WPI_DashboardDecode Status Byte.vi"("Window Mode Notifier"=w186, "Status"=w188) -> ("Mode"=→"Mode":T9)  [unwired: 1 out]
    n102 = case shown="\"0.0.0.0\"" w181 {
      selector: w181 -> [_ w208]
      tunnel: w182 -> [_ w209]
      tunnel: w180 -> [_ _]
      tunnel: w179 -> [_ _]
      tunnel: w178 -> [_ _]
      tunnel: w177 -> [_ w207]
      frame "0.0.0.0" {
        # "DS not sending packets, or no robot exists yet.\nDon't poll the variables"
      }
      frame Default {
        # "Notify NT\nBind loop"
        # "DS sent a packet. use any data it\nprovided, poll others and update\ndisplays that don'teasily bind\nusing names"
        # "swap motors to match\ncharts and include battery"
        n103 = Send Notification(notification=w208, notifier=w209) -> ()  [unwired: 1 in, 2 out]
        n104 = call <vilib>:"SD Read Number.vi"("Name"="Gyro_Dist") -> ("Numeric"=w196:dbl)  [unwired: 8 in, 2 out]
        n105 = call <vilib>:"SD Read Numeric Array.vi"("Name"="RobotDrive Motors") -> ("Numeric Array"=w206:dbl[])  [unwired: 8 in, 2 out]
        n106 = call <vilib>:"SD Read String.vi"("Name"="ShooterstateDS") -> ("String"=w192:string)  [unwired: 8 in, 2 out]
        n107 = call <vilib>:"SD Read Number.vi"("Name"="Sonar_Dist") -> ("Numeric"=w194:dbl)  [unwired: 8 in, 2 out]
        n108 = call <vilib>:"SD Read Boolean.vi"("Name"="Compressor_Running") -> ("Boolean"=w190:bool)  [unwired: 8 in, 2 out]
        n109 = call <vilib>:"SD Read Numeric Array.vi"("Name"="Joystick 1/Axes") -> ("Numeric Array"=w225:dbl[])  [unwired: 8 in, 2 out]
        n110 = call <vilib>:"SD Read Boolean Array.vi"("Name"="Joystick 1/Buttons") -> ("Boolean Array"=w227:bool[])  [unwired: 8 in, 2 out]
        n111 = call <vilib>:"SD Read Numeric Array.vi"("Name"="Joystick 2/Axes") -> ("Numeric Array"=w219:dbl[])  [unwired: 8 in, 2 out]
        n112 = call <vilib>:"SD Read Boolean Array.vi"("Name"="Joystick 2/Buttons") -> ("Boolean Array"=w218:bool[])  [unwired: 8 in, 2 out]
        n113 = Index Array(array=w206, index #1=1, index #4=0) -> (element #1=w202:dbl, element #2=w201:dbl, element #3=w203:dbl, element #4=w198:dbl)  [unwired: 2 in]
        n114 = local write "Shooter_State"(w192) -> ()
        n115 = local write "sonar_ball_distance"(w194) -> ()
        n116 = Array To Cluster(array=w227) -> (cluster=→"JS Buttons 1":T26)
        n117 = Array To Cluster(array=w218) -> (cluster=→"JS Buttons 2":T26)
        n118 = local write "robot_heading"(w196) -> ()
        n119 = Index Array(array=w225) -> (element #1=w222:dbl, element #2=w223:dbl, element #3=→"JS1 Z":dbl)  [unwired: 6 in, 3 out]
        n120 = Index Array(array=w219) -> (element #1=w214:dbl, element #2=w213:dbl, element #3=→"JS2 Z":dbl)  [unwired: 3 in]
        n121 = local write "Compressor_Running"(w190) -> ()
        n122 = Bundle("Numeric"=w203, "Numeric"=w202) -> (→"MotorChart R" →"MotorSliders R":cluster{"Numeric":dbl, "Numeric":dbl})  [unwired: 1 in]
        n123 = Bundle("Numeric"=w201, "Numeric"=w198, "Battery"=w207) -> (→"MotorChart L" →"MotorSliders L":T7)  [unwired: 1 in]
        n124 = Bundle("Numeric"=w222, "Numeric"=w223) -> (w221:cluster{"Numeric":dbl, "Numeric":dbl})  [unwired: 1 in]
        n125 = Bundle("Numeric"=w214, "Numeric"=w213) -> (w215:cluster{"Numeric":dbl, "Numeric":dbl})  [unwired: 1 in]
        n126 = Build Array(w221) -> (→"Joystick 1":cluster{"Numeric":dbl, "Numeric":dbl}[])
        n127 = Build Array(w215) -> (→"Joystick 2":cluster{"Numeric":dbl, "Numeric":dbl}[])
      }
    }
  }
  n128 = while {
    tunnel: w3 -> [w241]
    tunnel: w29 -> [w239]
    tunnel: [w237] -> _
    tunnel: u32 1000 ("milliseconds to wait") -> [w236]
    i -> [w237]
    stop <- FALSE stop-if-true
    n129 = local read "Rec Mode"() -> (w232:enum32{"Stop", "Record", "Playback"})
    n130 = Wait on Notification(notifier=w239, timeout in ms (-1)=w236) -> (notification=w238:string, timed out?=w234:bool)  [unwired: 2 in, 2 out]
    n131 = Equal?(x=w232, y=u16 2 ("Rec Mode")) -> (x = y?=w233:bool)
    n132 = Compound Arithmetic op=OR(invert w234, w233) -> (w235:bool)
    n133 = case shown="False" w235 {
      tunnel: w241 -> [_ w243]
      tunnel: w238 -> [_ w242]
      frame False {
      }
      frame True {
        n134 = call <vilib>:"Bind Controls to SmartDashboard.vi"("Bound Control Refs"=w243, "Server IP Address"=w242) -> ()  [unwired: 10 in]
      }
    }
  }
  n135 = register-events(refnum<vi> refnum) -> (reference out=w16:refnum<event-registration>, error out=w15:errorcluster)  [unwired: 2 in]
  n136 = vi-ref "Playback Controls.vi"() -> (w17:refnum<vi>)
  n137 = call "Initialize Camera and CheckList.vi"("ListBox in"=w9) -> ("Cluster"=w23:cluster{"value":i32, "value":i32, "index":i32}, "Array"=w24:cluster{string[]}[], "File Refnum"=w22:T27)  [unwired: 8 in]
  n138 = property on="Camera Settings" class="Clust (strict)"("Val(Sgnl)"=w23) -> ()  [unwired: 2 in, 2 out]
  n139 = control-ref of="Test Tree"() -> (w21:refnum<vi>)
  n140 = while {
    tunnel: w24 -> [w251]
    shift-right: [w250] -> _
    shift-left: w22 -> [w249]
    tunnel: [w248] -> _
    tunnel: w21 -> [w247]
    tunnel: w17 -> [w246]
    tunnel: w16 -> [w245]
    tunnel: w15 -> [_]
    tunnel: w7 -> [w244]
    i -> [w248]
    stop <- FALSE stop-if-true
    n141 = event shown="[0] Timeout" {
      selector: w245 -> [_ _ _ _ _ _ _ _ _ _ _ _ _ _ _ _]
      dyn-events: [_ _ _ _ _ _ _ _ _ _ _ _ _ w489 _ _] -> _
      timeout: u32 60 ("milliseconds to wait") -> [_ _ _ _ _ _ _ _ _ _ _ _ _ _ _ _]
      tunnel: w247 -> [w261 _ _ _ _ _ _ _ _ _ _ _ _ _ _ _]
      tunnel: "Test Tree" -> [_ _ _ _ _ _ _ _ w458 w466 w468 w472 w480 _ _ _]
      tunnel: w251 -> [_ w285 _ _ _ _ w422 w452 _ _ _ _ _ _ _ _]
      tunnel: [w255 w284 w383 w388 w396 w408 w421 w445 w457 w464 w467 w471 w479 w491 w505 w506] -> w250
      tunnel: w249 -> [w255 w284 w383 w388 w396 w408 w420 w445 w457 w464 w467 w471 w479 w491 w505 w506]
      tunnel: w246 -> [_ _ _ _ _ _ _ _ _ _ _ _ _ w492 _ w509]
      tunnel: w244 -> [_ _ _ _ _ _ _ _ _ _ _ _ _ w487 _ _]
      event Timeout {
        w260 = enum16{"Update", "Clear"}[] [enum."Clear", enum."Clear", enum."Clear", enum."Clear", enum."Update", enum."Update", enum."Clear"] items=["Update", "Clear"]
        n142 = event-data() -> ()  [unwired: 1 in, 1 out]
        n143 = local read "Mode"() -> (w258:T9)
        n144 = Index Array(array=w260, index=w258) -> (element=w259:enum16{"Update", "Clear"})
        n145 = call <vilib>:"NT Read String.vi"("Name"="TestMode/TestName") -> ("String"=w264:string)  [unwired: 9 in, 1 out]
        n146 = case shown="\"Operation\", Default" "Dashboard Tab" {
          tunnel: w261 -> [_ w274 _]
          tunnel: "/TestMode/Automatic/" ("Name Pattern") -> [_ w273 _]
          tunnel: w259 -> [_ w272 _]
          tunnel: w258 -> [_ w270 _]
          tunnel: [_ _ w276] -> _
          frame "Operation", Default {
          }
          frame "Test" {
            w269 = -2 ("Active Item:Row Number")
            n147 = call <vilib>:"NT Read and Format Entries as Tree.vi"("Operation"=w272, "Name Pattern"=w273, "Tree Refnum"=w274) -> ()  [unwired: 7 in, 2 out]
            n148 = Index Array(array=u32[] [14013909, 14013909, 14013909, 14013909, 14013909, 16777215, 14013909], index=w270) -> (element=w268:u32)
            n149 = property on="Test Tree" class="Tree (strict)"("Active Item Row Number"=w269, "ActiveColNum"=w269, "CellBG"=w268, "Active Item Row Number"=-1 ("Active Item:Row Number"), "CellBG"=u32 5789784 ("Color Box")) -> ()  [unwired: 2 in, 2 out]
          }
          frame "Variables" {
            n150 = control-ref of="Tree"() -> (w275:refnum<vi>)
            n151 = call <vilib>:"NT Read and Format Entries as Tree.vi"("Tree Refnum"=w275) -> ("Formatted Strings"=w276:cluster{"Name":string, "Value":string}[])  [unwired: 9 in, 1 out]
          }
        }
        n152 = case shown="\"\"" w264 {
          tunnel: "TestMode/TestProgress" ("Name") -> [w278 _]
          tunnel: "TestMode/TestProgressText" ("Name") -> [w277 _]
          frame Default {
            n153 = call <vilib>:"NT Read Number.vi"("Name"=w278) -> ("Numeric"=w279:dbl)  [unwired: 9 in, 1 out]
            n154 = call <vilib>:"NT Read String.vi"("Name"=w277) -> ("String"=w280:string)  [unwired: 9 in, 1 out]
            n155 = Bundle("Numeric"=w279, "String"=w280) -> (→"Progress":cluster{"Numeric":dbl, "String":string})  [unwired: 1 in]
          }
          frame "" {
            n156 = property on="Progress" class="Clust (strict)"("Visible"=FALSE) -> ()  [unwired: 2 in, 2 out]
            n157 = local write "Test Name"(u16 0) -> ()
          }
        }
      }
      event "Test Tree": Value Change {
        # "Show appropriate\ncontrols"
        n158 = event-data() -> ("CtlRef"=w288:refnum<vi>, "NewVal"=w286:string)  [unwired: 1 in]
        n159 = call <vilib>:"WPI_UtilitiesGetTreeIOName.vi"("NewVal"=w286, "TreeControl in"=w288) -> ("I/O Name"=w289:string)  [unwired: 9 in]
        n160 = case shown="\"Camera\"" w289 {
          selector: w289 -> [_ w296 _ w314 w323 _]
          tunnel: w286 -> [_ _ w311 w313 _ w330]
          tunnel: w285 -> [_ _ _ _ _ w329]
          frame Default {
            w291 = FALSE ("Visible")
            w290 = FALSE ("Visible")
            n161 = property on="Motor" class="Clust (strict)"("Visible"=w290) -> ()  [unwired: 2 in, 2 out]
            n162 = property on="Test Ring" class="Ring (strict)"("Visible"=w290) -> ()  [unwired: 2 in, 2 out]
            n163 = property on="Rev/Fwd" class="Clust (strict)"("Visible"=w291) -> ()  [unwired: 2 in, 2 out]
            n164 = property on="On/Off" class="Bool (strict)"("Visible"=w291) -> ()  [unwired: 2 in, 2 out]
            n165 = property on="Test Slider" class="Slide (strict)"("Visible"=w291) -> ()  [unwired: 2 in, 2 out]
          }
          frame "Motor", "PWM" {
            w297 = FALSE ("Visible")
            n166 = case shown="\"Motor\", Default" w296 {
              tunnel: [1.0 ("Value") -1.0 ("Value")] -> w295
              tunnel: [255.0 ("Value") 1.0 ("Value")] -> w294
              tunnel: [128.0 ("Value") 0.0 ("Value")] -> w293
              tunnel: [64.0 ("Value") 0.5 ("Value")] -> w292
              frame "PWM" {
              }
              frame "Motor", Default {
              }
            }
            n167 = property on="Motor" class="Clust (strict)"("Visible"=TRUE) -> ()  [unwired: 2 in, 2 out]
            n168 = property on="Value" class="Slide (strict)"("Value"=w293, "Scale.Minimum"=w295, "Scale.Maximum"=w294, "Scale.Increment"=w292) -> ()  [unwired: 2 in, 2 out]
            n169 = property on="On/Off" class="Bool (strict)"("Visible"=w297) -> ()  [unwired: 2 in, 2 out]
            n170 = property on="Test Slider" class="Slide (strict)"("Visible"=w297) -> ()  [unwired: 2 in, 2 out]
            n171 = property on="Test Ring" class="Ring (strict)"("Visible"=w297) -> ()  [unwired: 2 in, 2 out]
            n172 = property on="Rev/Fwd" class="Clust (strict)"("Visible"=w297) -> ()  [unwired: 2 in, 2 out]
          }
          frame "Servo" {
            w309 = FALSE ("Visible")
            n173 = call <vilib>:"NT Read Number.vi"("Name"=w311) -> ("Numeric"=w310:dbl)  [unwired: 9 in, 1 out]
            n174 = property on="Test Slider" class="Slide (strict)"("Visible"=TRUE, "Scale.Maximum"=170.0 ("Scale.Range:Maximum")) -> ()  [unwired: 2 in, 2 out]
            n175 = local write "Test Slider"(w310) -> ()
            n176 = property on="Motor" class="Clust (strict)"("Visible"=w309) -> ()  [unwired: 2 in, 2 out]
            n177 = property on="Rev/Fwd" class="Clust (strict)"("Visible"=w309) -> ()  [unwired: 2 in, 2 out]
            n178 = property on="On/Off" class="Bool (strict)"("Visible"=w309) -> ()  [unwired: 2 in, 2 out]
            n179 = property on="Test Ring" class="Ring (strict)"("Visible"=w309) -> ()  [unwired: 2 in, 2 out]
          }
          frame "Relay", "Solenoid" {
            w312 = FALSE ("Visible")
            n180 = property on="Motor" class="Clust (strict)"("Visible"=w312) -> ()  [unwired: 2 in, 2 out]
            n181 = property on="Test Slider" class="Slide (strict)"("Visible"=w312) -> ()  [unwired: 2 in, 2 out]
            n182 = Search and Replace String(input string=w313, search string="/Value  **", replace string="/Direction") -> (result string=w319:string)  [unwired: 5 in, 3 out]
            n183 = property on="Test Ring" class="Ring (strict)"("Visible"=w312) -> ()  [unwired: 2 in, 2 out]
            n184 = call <vilib>:"NT Read String.vi"("Name"=w319) -> ("String"=w317:string)  [unwired: 9 in, 1 out]
            n185 = Equal?(x="Both directions", y=w317) -> (x = y?=w315:bool)
            n186 = Not(x=w315) -> (.not. x?=w316:bool)
            n187 = property on="Rev/Fwd" class="Clust (strict)"("Visible"=w315) -> ()  [unwired: 2 in, 2 out]
            n188 = property on="On/Off" class="Bool (strict)"("Visible"=w316, "Caption.Text"=w314) -> ()  [unwired: 2 in, 2 out]
          }
          frame "Compressor", "Digital Out" {
            w322 = FALSE ("Visible")
            # "Get direction and finish"
            n189 = property on="Motor" class="Clust (strict)"("Visible"=w322) -> ()  [unwired: 2 in, 2 out]
            n190 = property on="Test Slider" class="Slide (strict)"("Visible"=w322) -> ()  [unwired: 2 in, 2 out]
            n191 = property on="Test Ring" class="Ring (strict)"("Visible"=w322) -> ()  [unwired: 2 in, 2 out]
            n192 = property on="On/Off" class="Bool (strict)"("Visible"=TRUE, "Caption.Text"=w323) -> ()  [unwired: 2 in, 2 out]
            n193 = property on="Rev/Fwd" class="Clust (strict)"("Visible"=FALSE) -> ()  [unwired: 2 in, 2 out]
          }
          frame "Camera" {
            n194 = call <vilib>:"Get Last Path Segment.vi"("String in"=w330) -> ("String out"=w331:string)  [unwired: 10 in]
            n195 = property on="On/Off" class="Bool (strict)"("Visible"=FALSE) -> ()  [unwired: 2 in, 2 out]
            n196 = property on="Motor" class="Clust (strict)"("Visible"=FALSE) -> ()  [unwired: 2 in, 2 out]
            n197 = property on="Rev/Fwd" class="Clust (strict)"("Visible"=FALSE) -> ()  [unwired: 2 in, 2 out]
            n198 = case shown="\"White Balance  **\"" w331 {
              tunnel: w330 -> [w337 w346 w355 w364 w373 _ w379]
              tunnel: w329 -> [w335 w343 w352 w361 w370 _ _]
              frame "Size  **" {
                n199 = Index Array(array=w335) -> (element=w334:cluster{string[]})  [unwired: 1 in]
                n200 = call <vilib>:"NT Read String.vi"("Name"=w337) -> ("String"=w336:string)  [unwired: 9 in, 1 out]
                n201 = Unbundle(w334) -> (w332:string[])
                n202 = Match First String(2:w332, 3:w336) -> (0:w333:i32)  [unwired: 1 out]
                n203 = property on="Test Ring" class="Ring (strict)"("Value"=w333, "Strings []"=w332) -> ()  [unwired: 2 in, 2 out]
                n204 = property on="Test Ring" class="Ring (strict)"("Visible"=TRUE) -> ()  [unwired: 2 in, 2 out]
                n205 = property on="Test Slider" class="Slide (strict)"("Visible"=FALSE) -> ()  [unwired: 2 in, 2 out]
              }
              frame "White Balance  **" {
                n206 = Index Array(array=w343, index=1) -> (element=w344:cluster{string[]})
                n207 = call <vilib>:"NT Read String.vi"("Name"=w346) -> ("String"=w345:string)  [unwired: 9 in, 1 out]
                n208 = Unbundle(w344) -> (w341:string[])
                n209 = Match First String(2:w341, 3:w345) -> (0:w340:i32)  [unwired: 1 out]
                n210 = property on="Test Ring" class="Ring (strict)"("Value"=w340, "Strings []"=w341) -> ()  [unwired: 2 in, 2 out]
                n211 = property on="Test Ring" class="Ring (strict)"("Visible"=TRUE) -> ()  [unwired: 2 in, 2 out]
                n212 = property on="Test Slider" class="Slide (strict)"("Visible"=FALSE) -> ()  [unwired: 2 in, 2 out]
              }
              frame "Exposure  **" {
                n213 = Index Array(array=w352, index=2) -> (element=w353:cluster{string[]})
                n214 = call <vilib>:"NT Read String.vi"("Name"=w355) -> ("String"=w354:string)  [unwired: 9 in, 1 out]
                n215 = Unbundle(w353) -> (w349:string[])
                n216 = Match First String(2:w349, 3:w354) -> (0:w350:i32)  [unwired: 1 out]
                n217 = property on="Test Ring" class="Ring (strict)"("Value"=w350, "Strings []"=w349) -> ()  [unwired: 2 in, 2 out]
                n218 = property on="Test Ring" class="Ring (strict)"("Visible"=TRUE) -> ()  [unwired: 2 in, 2 out]
                n219 = property on="Test Slider" class="Slide (strict)"("Visible"=FALSE) -> ()  [unwired: 2 in, 2 out]
              }
              frame "Exposure Priority  **" {
                n220 = Index Array(array=w361, index=3) -> (element=w362:cluster{string[]})
                n221 = call <vilib>:"NT Read String.vi"("Name"=w364) -> ("String"=w363:string)  [unwired: 9 in, 1 out]
                n222 = Unbundle(w362) -> (w358:string[])
                n223 = Match First String(2:w358, 3:w363) -> (0:w359:i32)  [unwired: 1 out]
                n224 = property on="Test Ring" class="Ring (strict)"("Value"=w359, "Strings []"=w358) -> ()  [unwired: 2 in, 2 out]
                n225 = property on="Test Ring" class="Ring (strict)"("Visible"=TRUE) -> ()  [unwired: 2 in, 2 out]
                n226 = property on="Test Slider" class="Slide (strict)"("Visible"=FALSE) -> ()  [unwired: 2 in, 2 out]
              }
              frame "Color Enable  **" {
                n227 = Index Array(array=w370, index=4) -> (element=w371:cluster{string[]})
                n228 = call <vilib>:"NT Read String.vi"("Name"=w373) -> ("String"=w372:string)  [unwired: 9 in, 1 out]
                n229 = Unbundle(w371) -> (w367:string[])
                n230 = Match First String(2:w367, 3:w372) -> (0:w368:i32)  [unwired: 1 out]
                n231 = property on="Test Ring" class="Ring (strict)"("Value"=w368, "Strings []"=w367) -> ()  [unwired: 2 in, 2 out]
                n232 = property on="Test Ring" class="Ring (strict)"("Visible"=TRUE) -> ()  [unwired: 2 in, 2 out]
                n233 = property on="Test Slider" class="Slide (strict)"("Visible"=FALSE) -> ()  [unwired: 2 in, 2 out]
              }
              frame Default {
                n234 = property on="Test Ring" class="Ring (strict)"("Visible"=FALSE) -> ()  [unwired: 2 in, 2 out]
                n235 = property on="Test Slider" class="Slide (strict)"("Visible"=FALSE) -> ()  [unwired: 2 in, 2 out]
              }
              frame "Brightness  **", "Color Level  **", "Compression  **", "FPS  **", "Sharpness  **" {
                n236 = call <vilib>:"NT Read Number.vi"("Name"=w379) -> ("Numeric"=w378:dbl)  [unwired: 9 in, 1 out]
                n237 = local write "Test Slider"(w378) -> ()
                n238 = property on="Test Slider" class="Slide (strict)"("Visible"=TRUE, "Scale.Maximum"=100.0 ("Scale.Range:Maximum")) -> ()  [unwired: 2 in, 2 out]
                n239 = property on="Test Ring" class="Ring (strict)"("Visible"=FALSE) -> ()  [unwired: 2 in, 2 out]
              }
            }
          }
        }
        n240 = property on="Progress" class="Clust (strict)"("Visible"=FALSE) -> ()  [unwired: 2 in, 2 out]
      }
      event "Test Name": Mouse Enter {
        # "Populate the ring with the list of tests"
        n241 = event-data() -> ()  [unwired: 1 in, 1 out]
        n242 = call <vilib>:"NT Read String Array.vi"("Name"="TestMode/TestList") -> ("String Array"=w387:string[])  [unwired: 9 in, 1 out]
        n243 = Build Array (concatenate)("Select the test to run...", w387) -> (w386:string[])
        n244 = property on="Test Name" class="Ring (strict)"("Strings []"=w386) -> ()  [unwired: 2 in, 2 out]
      }
      event "Test Name": Value Change {
        w389 = FALSE ("Visible")
        # "Tell the robot the test name to run"
        n245 = event-data() -> ("NewVal"=w393:u16)  [unwired: 1 in]
        n246 = property on="Test Name" class="Ring (strict)"() -> ("Strings []"=w394:string[])  [unwired: 2 in, 2 out]
        n247 = local write "Progress"(T11 {"Test Progress"=0, "Test Progress Text"=""} ("Progress")) -> ()
        n248 = Index Array(array=w394, index=w393) -> (element=w392:string)
        n249 = call <vilib>:"NT Write String.vi"("String"=w392, "Name"="TestMode/TestName") -> ()  [unwired: 9 in, 1 out]
        n250 = property on="Progress" class="Clust (strict)"("Visible"=TRUE) -> ()  [unwired: 2 in, 2 out]
        n251 = property on="Motor" class="Clust (strict)"("Visible"=w389) -> ()  [unwired: 2 in, 2 out]
        n252 = property on="Test Slider" class="Slide (strict)"("Visible"=w389) -> ()  [unwired: 2 in, 2 out]
        n253 = property on="On/Off" class="Bool (strict)"("Visible"=w389) -> ()  [unwired: 2 in, 2 out]
        n254 = property on="Rev/Fwd" class="Clust (strict)"("Visible"=w389) -> ()  [unwired: 2 in, 2 out]
        n255 = property on="Test Ring" class="Ring (strict)"("Visible"=w389) -> ()  [unwired: 2 in, 2 out]
      }
      event "Listbox": Double Click {
        n256 = event-data() -> ("PlatMods.Shift"=w397:bool, "Row"=w399:i32)  [unwired: 1 in]
        n257 = case shown="True" w397 {
          tunnel: w399 -> [w403 _]
          tunnel: 1 -> [w402 _]
          frame False {
            n258 = property on="Listbox" class="LstBox (strict)"() -> ("Item Symbols"=w401:i32[])  [unwired: 2 in, 2 out]
            n259 = Replace Array Subset(array=w401, new element=w402, index=w403) -> (w400:i32[])
            n260 = property on="Listbox" class="LstBox (strict)"("Item Symbols"=w400) -> ()  [unwired: 2 in, 2 out]
          }
          frame True {
            w404 = 0 ("Top Row")
            n261 = property on="Listbox" class="LstBox (strict)"() -> ("Number of Rows"=w406:u32)  [unwired: 2 in, 2 out]
            n262 = Initialize Array(0, w406) -> (w405:i32[])
            n263 = property on="Listbox" class="LstBox (strict)"("Top Row"=w404, "Value"=w404, "Item Symbols"=w405) -> ()  [unwired: 2 in, 2 out]
          }
        }
      }
      event "Listbox": Key Down {
        n264 = event-data() -> ("VKey"=w410:T28)  [unwired: 1 in]
        n265 = case shown="\"Left\", \"Right\"" w410 {
          selector: w410 -> [w415 _]
          tunnel: eventvkey."Left" ("VKey") -> [w413 _]
          frame "Left", "Right" {
            n266 = Equal?(x=w413, y=w415) -> (x = y?=w414:bool)
            n267 = Select(t=0, s=w414, f=1) -> (s? t:f=w416:i32)
            n268 = property on="Listbox" class="LstBox (strict)"() -> ("Item Symbols"=w419:i32[])  [unwired: 2 in, 2 out]
            n269 = Replace Array Subset(array=w419, new element=w416, index="Listbox") -> (w418:i32[])
            n270 = property on="Listbox" class="LstBox (strict)"("Item Symbols"=w418) -> ()  [unwired: 2 in, 2 out]
          }
          frame Default {
          }
        }
      }
      event "DB Camera Config": Value Change {
        n271 = event-data() -> ("NewVal"=w423:bool)  [unwired: 1 in]
        n272 = case shown="False" w423 {
          tunnel: w422 -> [w432 _]
          tunnel: [w425 w443] -> w421
          tunnel: w420 -> [w424 w443]
          frame False {
            w439 = "Camera"
            w442 = FALSE ("Visible")
            n273 = local read "Camera Settings"() -> (w431:T4)
            n274 = Index Array(array=w432) -> (element=w435:cluster{string[]})  [unwired: 1 in]
            n275 = Unbundle(w431) -> ("Frame Rate"=w430:i32, "Compression"=w429:i32, "Size"=w433:u16)
            n276 = Unbundle(w435) -> (w434:string[])
            n277 = Index Array(array=w434, index=w433) -> (element=w428:string)
            n278 = call-poly <vilib>:"Write Key.vi"("section"=w439, "value"=w428, "key"="Size", "refnum"=w424) -> ("refnum out"=w441:T27)  [unwired: 2 in, 5 out]
            n279 = call-poly <vilib>:"Write Key.vi"("section"=w439, "value"=w430, "key"="FrameRate", "refnum"=w441) -> ("refnum out"=w440:T27)  [unwired: 1 in, 6 out]
            n280 = property on="Camera Settings" class="Clust (strict)"("Visible"=w442) -> ()  [unwired: 2 in, 2 out]
            n281 = local write "DB Camera Config"(w442) -> ()
            n282 = call-poly <vilib>:"Write Key.vi"("section"=w439, "value"=w429, "key"="Compression", "refnum"=w440) -> ("refnum out"=w426:T27)  [unwired: 1 in, 6 out]
            n283 = call <vilib>:"Close Config Data.vi"("refnum"=w426) -> ("file path"=w427:path)  [unwired: 2 in, 8 out]
            n284 = call <vilib>:"Open Config Data.vi"("configuration file path"=w427) -> ("refnum"=w425:T27)  [unwired: 8 in, 2 out]
          }
          frame True {
            n285 = property on="Camera Settings" class="Clust (strict)"("Visible"=TRUE) -> ()  [unwired: 2 in, 2 out]
          }
        }
      }
      event "Camera Settings": Value Change {
        n286 = event-data() -> ("NewVal"=w456:T4)  [unwired: 1 in]
        n287 = Index Array(array=w452) -> (element=w451:cluster{string[]})  [unwired: 1 in]
        n288 = Unbundle(w456) -> ("Frame Rate"=w447:i32, "Compression"=w446:i32, "Size"=w449:u16)
        n289 = Unbundle(w451) -> (w450:string[])
        n290 = Index Array(array=w450, index=w449) -> (element=w448:string)
        n291 = Format Into String(format string="%s   %dfps   %d%%", w448, w447, w446) -> (resulting string=w453:string)  [unwired: 2 in, 1 out]
        n292 = Build Array(w453) -> (w454:string[])
        n293 = property on="DB Camera Config" class="Bool (strict)"("Strings [4]"=w454) -> ()  [unwired: 2 in, 2 out]
      }
      event "Motor.Enable": Value Change {
        n294 = event-data() -> ("NewVal"=w462:bool)  [unwired: 1 in]
        n295 = Unbundle("Motor") -> ("Value"=w461:dbl)  [unwired: 1 out]
        n296 = Select(t=w461, s=w462, f=0.0) -> (s? t:f=w459:dbl)
        n297 = call <vilib>:"NT Write Number.vi"("Numeric"=w459, "Name"=w458) -> ()  [unwired: 9 in, 1 out]
      }
      event "Test Slider": Value Change {
        n298 = event-data() -> ("NewVal"=w465:dbl)  [unwired: 1 in]
        n299 = call <vilib>:"NT Write Number.vi"("Numeric"=w465, "Name"=w466) -> ()  [unwired: 9 in, 1 out]
      }
      event "On/Off": Value Change {
        n300 = event-data() -> ("NewVal"=w470:bool)  [unwired: 1 in]
        n301 = Boolean To (0,1)(Boolean=w470) -> (0, 1=w469:i16)
        n302 = call <vilib>:"NT Write Number.vi"("Numeric"=w469, "Name"=w468) -> ()  [unwired: 9 in, 1 out]
      }
      event "Rev/Fwd": Value Change {
        n303 = event-data() -> ("NewVal.Forward"=w478:bool, "NewVal.Reverse"=w477:bool)  [unwired: 1 in]
        n304 = Boolean To (0,1)(Boolean=w478) -> (0, 1=w474:i16)
        n305 = Boolean To (0,1)(Boolean=w477) -> (0, 1=w476:i16)
        n306 = Negate(x=w476) -> (-x=w475:i16)
        n307 = Add(x=w474, y=w475) -> (x+y=w473:i16)
        n308 = call <vilib>:"NT Write Number.vi"("Numeric"=w473, "Name"=w472) -> ()  [unwired: 9 in, 1 out]
      }
      event "Test Ring": Value Change {
        n309 = event-data() -> ("NewVal"=w482:u16)  [unwired: 1 in]
        n310 = property on="Test Ring" class="Ring (strict)"() -> ("Strings []"=w483:string[])  [unwired: 2 in, 2 out]
        n311 = Index Array(array=w483, index=w482) -> (element=w481:string)
        n312 = call <vilib>:"NT Write String.vi"("String"=w481, "Name"=w480) -> ()  [unwired: 9 in, 1 out]
      }
      event "Rec Mode": Value Change {
        # "Update globals for recording mode and path to read log from.\nClear when logging and let NetworkTables set path for vision to\nuse."
        n313 = event-data() -> ("NewVal"=w493:enum32{"Stop", "Record", "Playback"})  [unwired: 1 in]
        n314 = global write "WPI_DashboardLogging Global.vi" "Logging Filename"(path "") -> ()
        n315 = case shown="\"Stop\", \"Record\"" w493 {
          tunnel: w492 -> [_ w495 w503]
          tunnel: [_ _ w502] -> w489
          tunnel: [_ _ w501] -> _
          tunnel: w487 -> [_ _ w499]
          tunnel: cluster{i32, i32} {-250, 170} -> [_ _ w498]
          tunnel: [_ _ T29 {"Image Size"=TRUE, "Image Type"=TRUE, "Pixel Value"=TRUE, "ROI Information"=TRUE, "Zoom Factor"=FALSE} ("Image Information Shown:All Elements")] -> w485
          tunnel: [_ _ TRUE ("Zoom Factor")] -> w484
          frame Default {
          }
          frame "Stop", "Record" {
            # "Place Window too"
            n316 = invoke class="VI" method="FP.Close"(reference=w495) -> (reference out=w494:refnum<vi>)  [unwired: 2 in, 2 out]
            n317 = invoke class="VI" method="Abort VI"(reference=w494) -> ()  [unwired: 2 in, 3 out]
          }
          frame "Playback" {
            n318 = call "Open Playback Panel.vi"("Offset"=w498, "DB VI Ref"=w499, "Playback in"=w503) -> ("Playback out"=w500:refnum<vi>)  [unwired: 8 in]
            n319 = register-events(w500) -> (reference out=w502:refnum<event-registration>, error out=w501:errorcluster)  [unwired: 2 in]
          }
        }
        n320 = global write "WPI_DashboardLogging Global.vi" "Recording"(w493) -> ()
        n321 = property on="Camera Image" class="ImageControl"("Image Information Shown"=w485, "Image Information Visible"=w484) -> ()  [unwired: 2 in, 2 out]
        n322 = call <vilib>:"WPI_DashboardNT Log FieldName Cache.vi"("Operation"=enum16{"Lookup/Add", "Index", "Clear"}."Clear") -> ()  [unwired: 8 in, 3 out]
      }
      event Panel Close {
        w504 = enum32{"Stop", "Record", "Playback"}."Stop" ("Rec Mode")
        n323 = event-data() -> ()  [unwired: 1 in, 4 out]
        n324 = local write "Rec Mode"(w504) -> ()
        n325 = global write "WPI_DashboardLogging Global.vi" "Recording"(w504) -> ()
      }
      event Panel Close {
        # "Abort playback window and ourself"
        n326 = event-data() -> ()  [unwired: 1 in, 4 out]
        n327 = invoke class="VI" method="FP.Close"(reference=w509) -> (reference out=w508:refnum<vi>)  [unwired: 2 in, 2 out]
        n328 = invoke class="VI" method="Abort VI"(reference=w508) -> (error out=w507:errorcluster)  [unwired: 2 in, 2 out]
        n329 = invoke class="VI" method="Abort VI"(error in=w507) -> ()  [unwired: 2 in, 3 out]
      }
    }
  }
  n330 = property on="On/Off" class="Bool (strict)"("Visible"=w25) -> ()  [unwired: 2 in, 2 out]
  n331 = property on="Motor" class="Clust (strict)"("Visible"=w25) -> ()  [unwired: 2 in, 2 out]
  n332 = property on="Progress" class="Clust (strict)"("Visible"=w25) -> ()  [unwired: 2 in, 2 out]
  n333 = property on="Test Ring" class="Ring (strict)"("Visible"=w25) -> ()  [unwired: 2 in, 2 out]
  n334 = property on="Rev/Fwd" class="Clust (strict)"("Visible"=w25) -> ()  [unwired: 2 in, 2 out]
  n335 = property on="Camera Settings" class="Clust (strict)"("Visible"=w25) -> ()  [unwired: 2 in, 2 out]
  n336 = local write "DB Camera Config"(w25) -> ()
  n337 = global write "WPI_DashboardLogging Global.vi" "Recording"(w8) -> ()
  n338 = local write "Rec Mode"(w8) -> ()
